vi "Returning Values By Reference Simple Struct.vi"(7 "largerCircle":cluster{"x":sgl, "y":sgl, "radius":sgl}, 9 "radius":sgl, 10 "y":sgl, 11 "x":sgl) -> (5 "largerCircle out":cluster{"x":sgl, "y":sgl, "radius":sgl})   [LabVIEW 2018, in "ParsingDataSampleDLL.lvlib"]
doc: "__declspec(dllexport) void ReturningValuesByReference_SimpleStruct (struct simpleStructCircle circle, struct simpleStructCircle *largerCircle);"
uses:
  ParsingDataSampleDLL.lvlib
  ni_reference_vs/Debug/ParsingDataSampleDLL.dll
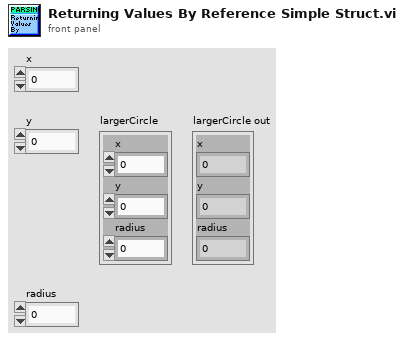
[diagram p1: front panel]
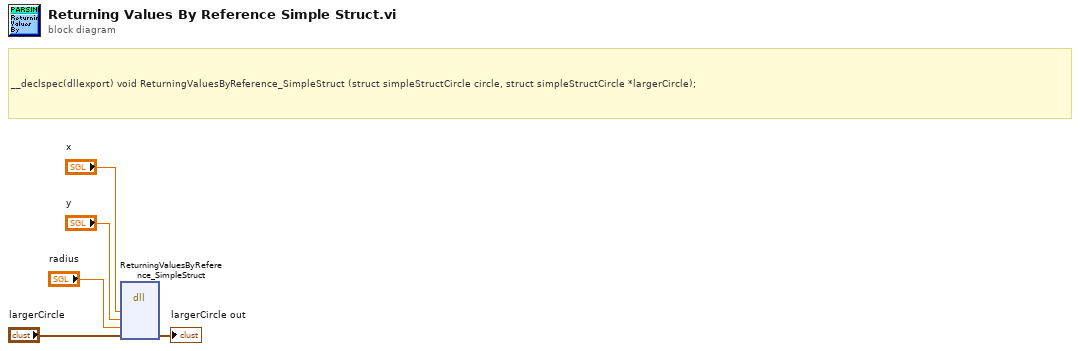
[diagram p0: block diagram]
diagram:
  # "__declspec(dllexport) void ReturningValuesByReference_SimpleStruct (struct simpleStructCircle circle, struct simpleStructCircle *largerCircle);"
  n1 = dll-call lib="C:/Users/celit/Documents/GitHub/Labview_Python_DLL_Call/ni_reference_vs/Debug/ParsingDataSampleDLL.*" fn="ReturningValuesByReference_SimpleStruct"("x"="x", "y"="y", "radius"="radius", "largerCircle"="largerCircle") -> ("largerCircle"=→"largerCircle out":cluster{"x":sgl, "y":sgl, "radius":sgl})  [unwired: 7 in, 2 out]
